vi "Do_ADAM_channel.vi"(4 "Scan Period":dbl format="%.2f", 5 "Previous Scan Value":dbl format="%.2f", 6 "Present scan array":dbl[](array[numeric]) format="%.2f", 7 "Value to Output":dbl format="%.2f", 8 "Ch Description":T1 {"Duty" format="%.0b"; "D" format="%#_5g"; "C" format="%#_5g"; "B" format="%#_5g"; "A" format="%#_5g"}, 9 "Ch names":string[](array[string])) -> (0 "Scan comment":string, 1 "Output":dbl format="%.3f")   [LabVIEW 2011]
uses:
  ADAM Client/Sub VIs/ADAM Controls/Ch_description_ADAM.ctl
  ADAM Client/Sub VIs/ADAM Controls/Module_type_ADAM.ctl
  ADAM Client/Sub VIs/ADAM Controls/Function_ADAM.ctl
  ADAM Client/Sub VIs/ADAM Controls/Channel_State.ctl
  ADAM Client/Sub VIs/ADAM Controls/Calib_type_ADAM.ctl
  ADAM Client/Sub VIs/ADAM Controls/Address.ctl
  ADAM Client/Sub VIs/ADAM Controls/Remember_value_mode.ctl
  ADAM Client/Sub VIs/ADAM Controls/Search_mode.ctl
  Anemometry/Anemometry Sub Vis/Controls/In_Range.ctl
  Anemometry/Anemometry Sub Vis/Globals/Gas_management_global.vi
  ADAM_Global.vi
  Anemometry/Anemometry Sub Vis/Globals/Constants_global.vi
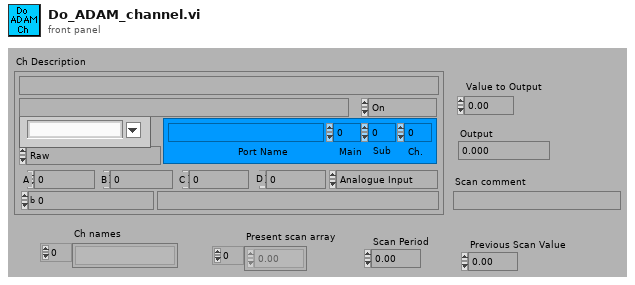
[diagram p1: front panel]
types:
  T1 = typedef "Ch_description_ADAM.ctl" = cluster{"Ch Name":string, "Type":T2, "Function":T3, "Ch State":T4, "Calibration type":T5, "A":dbl, "B":dbl, "C":dbl, "D":dbl, "Comments":string, "Address":T6, "String":string, "Duty":u16}
  T2 = typedef "Module_type_ADAM.ctl" = string
  T3 = typedef "Function_ADAM.ctl" = enum16{"Analogue Input", "Digital Input", "Event counter", "Event rate", "Analogue Output", "Digital Output", "Relay Output"}
  T4 = typedef "Channel_State.ctl" = enum16{"On", "Off", "Always On", "Always Off"}
  T5 = typedef "Calib_type_ADAM.ctl" = enum16{"Raw", "Bx + A", "Cx^2 + Bx + A", "Dx^3 + Cx^2 + Bx + A", "In Band", "Hi-Tec Q", "Hi-Tec M_dot", "Text"}
  T6 = typedef "Address.ctl" = cluster{"Main":i32, "Ch.":i32, "Sub":i32, "Port Name":string}
  T7 = typedef "Remember_value_mode.ctl" = enum16{"Read only", "Read and Write"}
  T8 = typedef "Search_mode.ctl" = enum16{"Between times", "All Times"}
  T9 = typedef "In_Range.ctl" = enum16{"%", "±", "% & ±"}
  T10 = typedef "Valco_valve_ph.ctl" = u16
  T11 = cluster{"Centre Times":dbl[], "Output array":dbl[]}
  T12 = cluster{"Centre Times":dbl[], "Output array":dbl[]}[]
  T13 = typedef "LVDateTimeRec.ctl" = cluster{"fractional second":dbl, "second":i32, "minute":i32, "hour":i32, "day of month":i32, "month":i32, "year":i32, "day of week":i32, "day of year":i32, "DST":i32}
  T14 = typedef "Client_State_Cluster.ctl" = cluster{"Client Name":string, "Traverse level State":T15, "People to Email":string[], "Next Contact Time":dbl}
  T15 = typedef "Traverse_Level_State.ctl" = enum16{"Running", "Complete"}
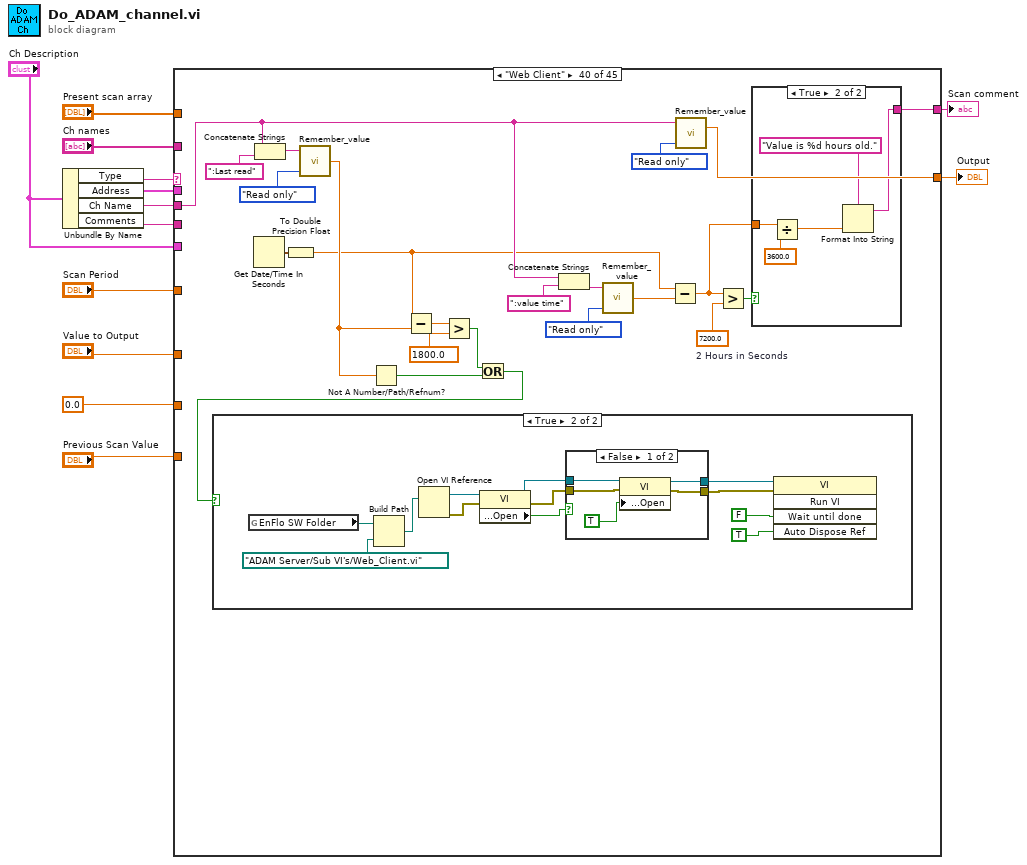
[diagram p0: block diagram]
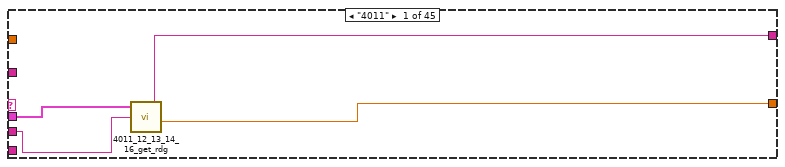
[diagram p2: hidden frame]
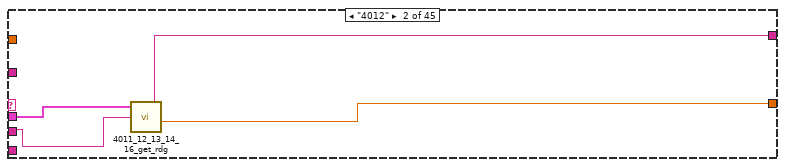
[diagram p3: hidden frame]
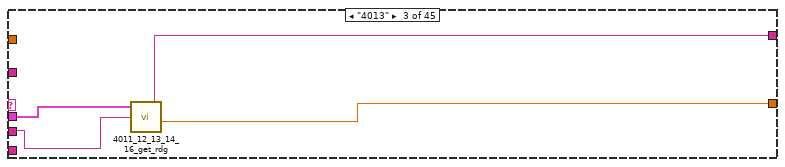
[diagram p4: hidden frame]
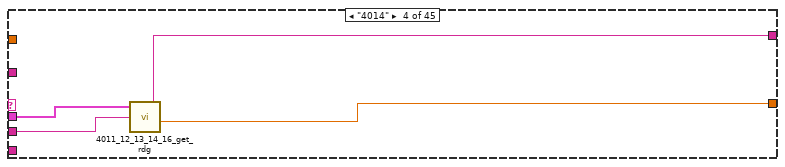
[diagram p5: hidden frame]
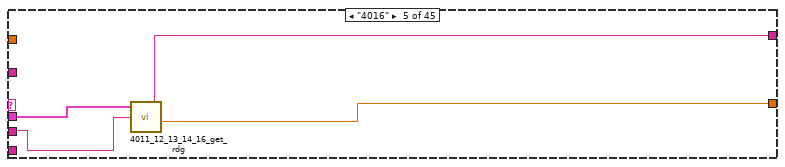
[diagram p6: hidden frame]
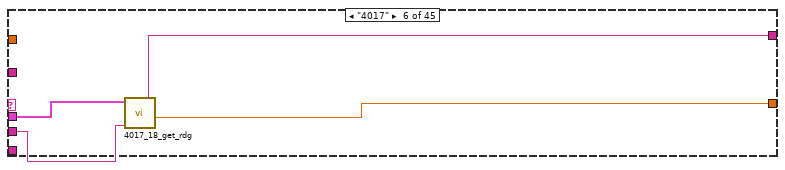
[diagram p7: hidden frame]
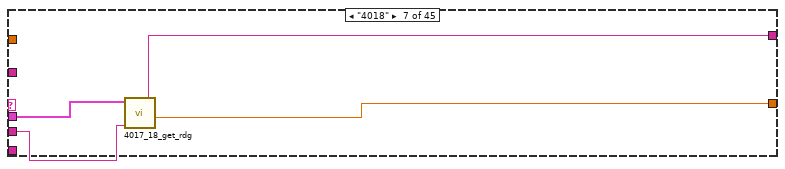
[diagram p8: hidden frame]
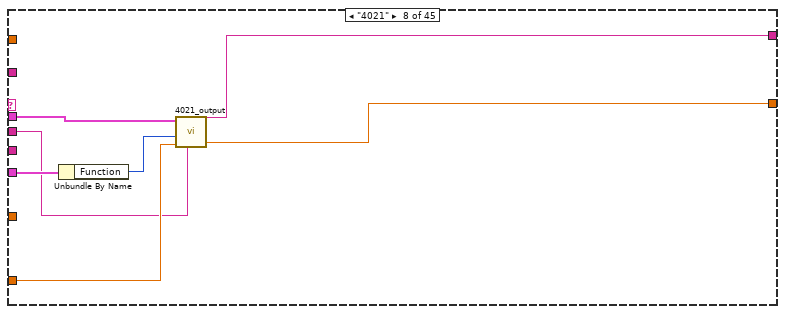
[diagram p9: hidden frame]
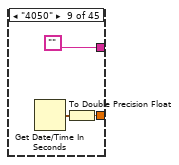
[diagram p10: hidden frame]
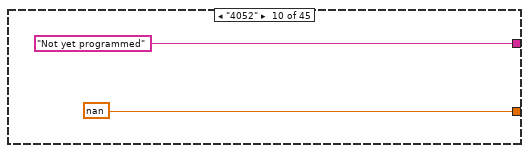
[diagram p11: hidden frame]
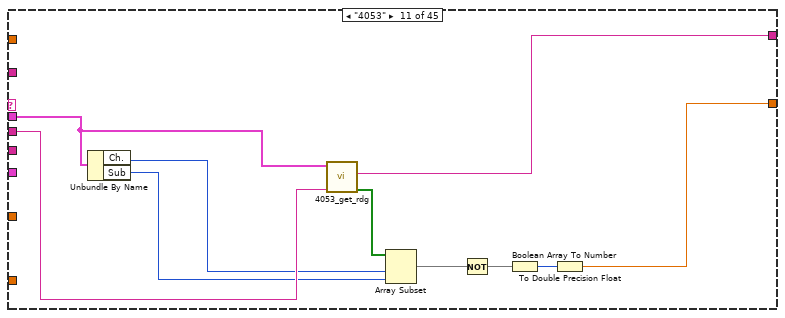
[diagram p12: hidden frame]
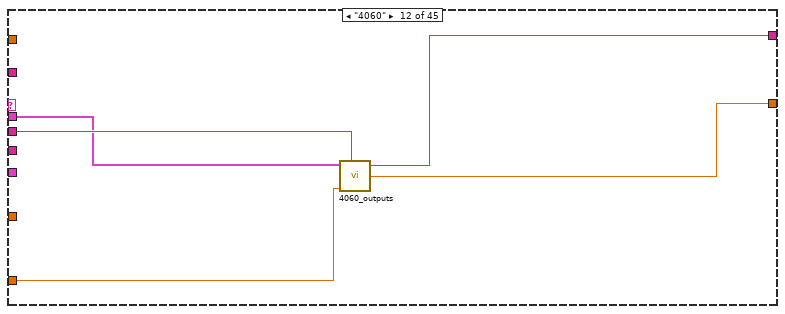
[diagram p13: hidden frame]
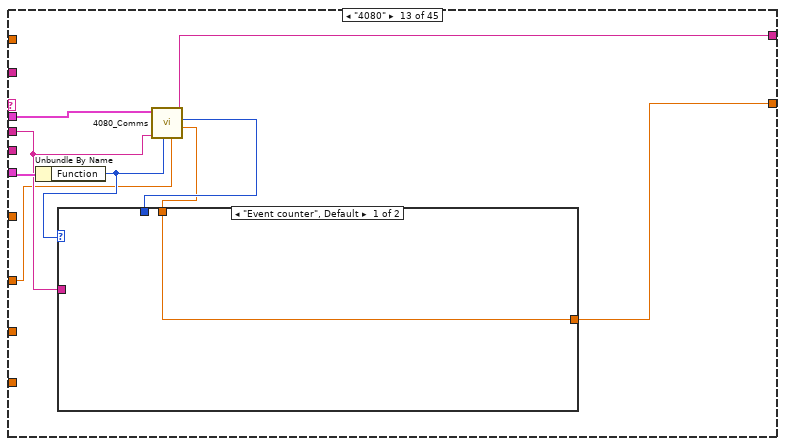
[diagram p14: hidden frame]
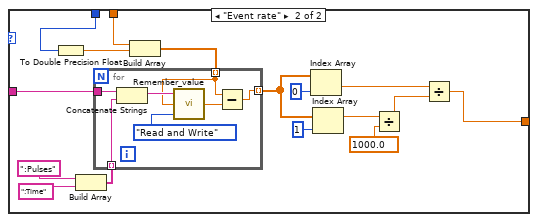
[diagram p15: hidden frame]
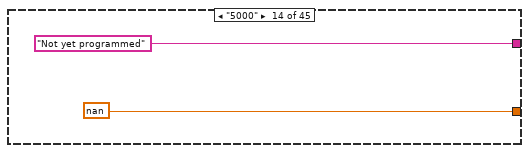
[diagram p16: hidden frame]
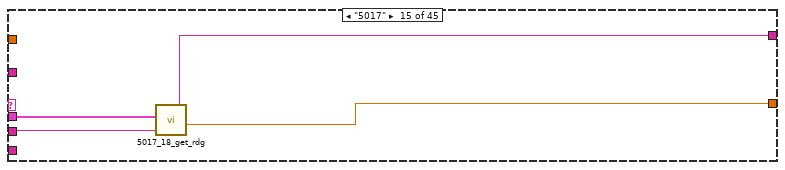
[diagram p17: hidden frame]
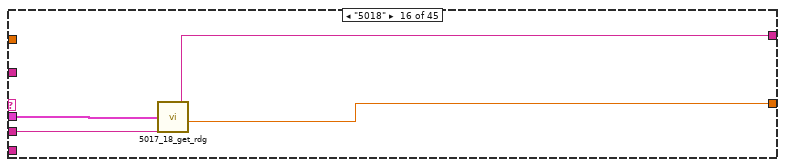
[diagram p18: hidden frame]
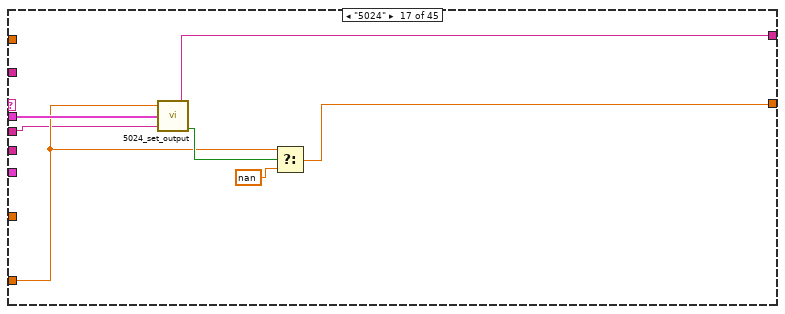
[diagram p19: hidden frame]
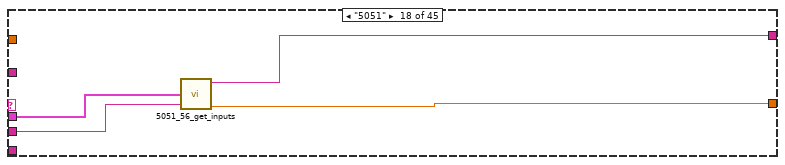
[diagram p20: hidden frame]
diagram:
  n1 = Unbundle By Name("Ch Description") -> ("Type"=w11:T2, "Address"=w10:T6, "Ch Name"=w2:string, "Comments"=w7:string)
  n2 = case shown="\"Web Client\"" w11 {
    tunnel: [w16 w20 w24 w28 w32 w36 w40 w47 w50 nan w57 w66 w75 nan w105 w109 w114 w120 w128 w149 w171 w190 nan w258 w260 w274 w299 w338 w348 w379 w384 w385 w497 w921 w923 w927 w932 nan ("Output") w946 w979 w1005 w1015 w1020 w1030 0.0 ("Output")] -> w8
    tunnel: [w17 w21 w25 w29 w33 w37 w41 w48 "" "Not yet programmed" w62 w67 w77 "Not yet programmed" w106 w110 w117 w121 w127 w150 w172 w192 "Not yet programmed" w257 w261 w273 w291 w339 w347 w380 w383 w406 w496 "" "" w928 "" "Not Yet Implemented" ("Status note") "" w968 "" w1016 w1019 "Crazy time based random number!" "Warning; unmatched case in Do_ADAM_channel" ("Status note")] -> w5
    tunnel: w10 -> [w14 w18 w22 w26 w30 w34 w38 w42 _ _ w54 w65 w69 _ w107 w111 w118 w122 w126 w151 w173 w194 _ w255 w259 w278 w296 w344 _ w378 w381 _ w488 _ _ _ _ _ _ _ w1014 w1018 _ _ _]
    tunnel: "Ch Description" -> [_ _ _ _ _ _ _ w46 _ _ _ _ w76 _ _ _ _ _ w125 w148 w170 w193 _ _ _ _ _ _ w353 _ _ w411 w490 _ w924 w929 _ _ _ _ _ _ w1021 _ _]
    tunnel: w2 -> [w15 w19 w23 w27 w31 w35 w39 w43 _ _ w63 w68 w72 _ w104 w108 w112 w119 w123 w145 w167 w191 _ w256 _ w276 w292 w343 _ _ w382 _ w493 _ _ _ _ _ w942 w975 _ w1017 _ _ _]
    tunnel: "Ch names" -> [_ _ _ _ _ _ _ _ _ _ _ _ _ _ _ _ _ _ _ _ _ _ _ _ _ _ _ _ w354 _ _ w410 w495 _ _ w930 _ _ _ _ _ _ _ _ _]
    tunnel: "Present scan array" -> [_ _ _ _ _ _ _ _ _ _ _ _ _ _ _ _ _ _ _ _ _ _ _ _ _ _ _ _ w351 _ _ w408 w494 _ _ w931 _ _ _ _ _ _ _ _ _]
    tunnel: w7 -> [_ _ _ _ _ _ _ _ _ _ _ _ _ _ _ _ _ _ _ _ _ _ _ _ _ _ _ _ w346 _ _ w412 _ _ _ _ _ _ _ _ _ _ _ _ _]
    tunnel: "Value to Output" -> [_ _ _ _ _ _ _ w44 _ _ _ w64 w70 _ _ _ w113 _ w124 w146 w168 w189 _ _ _ w262 w300 _ w352 _ _ _ _ _ _ _ _ _ _ _ w1009 _ _ _ _]
    tunnel: "Scan Period" -> [_ _ _ _ _ _ _ _ _ _ _ _ _ _ _ _ _ _ _ _ _ _ _ _ _ _ _ _ w349 _ _ _ w492 _ _ _ _ _ _ _ _ _ _ _ _]
    tunnel: "Previous Scan Value" -> [_ _ _ _ _ _ _ _ _ _ _ _ _ _ _ _ _ _ _ _ _ _ _ _ _ _ _ _ w350 _ _ w386 w491 w921 _ _ w932 _ _ _ _ _ _ _ _]
    tunnel: 0.0 -> [_ _ _ _ _ _ _ _ _ _ _ _ _ _ _ _ _ _ _ _ _ _ _ _ _ _ _ _ _ _ _ _ w489 _ _ _ _ _ _ _ _ _ _ _ _]
    frame "4011" {
      n3 = call "4011_12_13_14_16_get_rdg.vi"("Address"=w14, "Channel Name"=w15) -> ("Comment"=w17:string, "Reading"=w16:dbl)  [unwired: 1 in, 2 out]
    }
    frame "4012" {
      n4 = call "4011_12_13_14_16_get_rdg.vi"("Address"=w18, "Channel Name"=w19) -> ("Comment"=w21:string, "Reading"=w20:dbl)  [unwired: 1 in, 2 out]
    }
    frame "4013" {
      n5 = call "4011_12_13_14_16_get_rdg.vi"("Address"=w22, "Channel Name"=w23) -> ("Comment"=w25:string, "Reading"=w24:dbl)  [unwired: 1 in, 2 out]
    }
    frame "4014" {
      n6 = call "4011_12_13_14_16_get_rdg.vi"("Address"=w26, "Channel Name"=w27) -> ("Comment"=w29:string, "Reading"=w28:dbl)  [unwired: 1 in, 2 out]
    }
    frame "4016" {
      n7 = call "4011_12_13_14_16_get_rdg.vi"("Address"=w30, "Channel Name"=w31) -> ("Comment"=w33:string, "Reading"=w32:dbl)  [unwired: 1 in, 2 out]
    }
    frame "4017" {
      n8 = call "4017_18_get_rdg.vi"("Channel Name"=w35, "Address"=w34) -> ("Reading"=w36:dbl, "Comment"=w37:string)  [unwired: 2 in, 2 out]
    }
    frame "4018" {
      n9 = call "4017_18_get_rdg.vi"("Channel Name"=w39, "Address"=w38) -> ("Reading"=w40:dbl, "Comment"=w41:string)  [unwired: 2 in, 2 out]
    }
    frame "4021" {
      n10 = Unbundle By Name(w46) -> ("Function"=w45:T3)
      n11 = call "4021_output.vi"("Address"=w42, "Function"=w45, "Set to:"=w44, "Channel Name"=w43) -> ("Comment"=w48:string, "Reading"=w47:dbl)  [unwired: 1 in, 1 out]
    }
    frame "4050" {
      n12 = Get Date/Time In Seconds() -> (seconds since 1Jan1904=w49:timestamp)
      n13 = To Double Precision Float(number=w49) -> (double precision float=w50:dbl)
    }
    frame "4052" {
    }
    frame "4053" {
      n14 = Unbundle By Name(w54) -> ("Ch."=w55:i32, "Sub"=w61:i32)
      n15 = call "4053_get_rdg.vi"("Channel Name"=w63, "Address"=w54) -> ("Boolean array"=w60:bool[], "Comment"=w62:string)  [unwired: 2 in, 2 out]
      n16 = Array Subset(array=w60, index=w55, length=w61) -> (w59:bool[])
      n17 = Not(x=w59) -> (.not. x?=w56:bool[])
      n18 = Boolean Array To Number(Boolean array=w56) -> (number=w58:u32)
      n19 = To Double Precision Float(number=w58) -> (double precision float=w57:dbl)
    }
    frame "4060" {
      n20 = call "4060_outputs.vi"("Address"=w65, "Value to Output"=w64, "Channel Name"=w68) -> ("Comment"=w67:string, "Reading"=w66:dbl)  [unwired: 2 in, 1 out]
    }
    frame "4080" {
      n21 = Unbundle By Name(w76) -> ("Function"=w71:T3)
      n22 = call "4080_Comms.vi"("Value to display"=w70, "Function"=w71, "Channel Name"=w72, "Address"=w69) -> ("Reading"=w73:dbl, "millisecond timer value"=w74:u32, "Comment"=w77:string)  [unwired: 2 in, 1 out]
      n23 = case shown="\"Event counter\", Default" w71 {
        tunnel: w72 -> [_ w94]
        tunnel: w74 -> [_ w87]
        tunnel: [w78 w79] -> w75
        tunnel: w73 -> [w78 w88]
        frame "Event counter", Default {
        }
        frame "Event rate" {
          n24 = To Double Precision Float(number=w87) -> (double precision float=w86:dbl)
          n25 = Build Array(":Pulses", ":Time") -> (w89:string[])
          n26 = Build Array(w88, w86) -> (w85:dbl[])
          n27 = for {
            tunnel: w94 -> [w98]
            tunnel: [w99] -> w82 mode=indexing
            tunnel: w89 -> [w96] mode=indexing
            tunnel: w85 -> [w95] mode=indexing
            n28 = Concatenate Strings(w98, w96) -> (w97:string)
            n29 = call "Remember_value.vi"("Mode"=Remember_value_mode."Read and Write", "Input Value"=w95, "Ch name"=w97) -> ("Output Value"=w100:dbl)
            n30 = Subtract(x=w95, y=w100) -> (x-y=w99:dbl)
          }
          n31 = Index Array(array=w82, index=0) -> (element=w80:dbl)
          n32 = Index Array(array=w82, index=1) -> (element=w81:dbl)
          n33 = Divide(x=w81, y=1000.0) -> (x/y=w92:dbl)
          n34 = Divide(x=w80, y=w92) -> (x/y=w79:dbl)
        }
      }
    }
    frame "5000" {
    }
    frame "5017" {
      n35 = call "5017_18_get_rdg.vi"("Address (all reqd.)"=w107, "Channel Name"=w104) -> ("Comment"=w106:string, "Reading"=w105:dbl)  [unwired: 3 out]
    }
    frame "5018" {
      n36 = call "5017_18_get_rdg.vi"("Address (all reqd.)"=w111, "Channel Name"=w108) -> ("Comment"=w110:string, "Reading"=w109:dbl)  [unwired: 3 out]
    }
    frame "5024" {
      n37 = call "5024_set_output.vi"("Set to:"=w113, "Address (all reqd.)"=w118, "Channel Name"=w112) -> ("Comment"=w117:string, "Good Reply"=w115:bool)  [unwired: 2 out]
      n38 = Select(t=w113, s=w115, f=nan) -> (s? t:f=w114:dbl)
    }
    frame "5051" {
      n39 = call "5051_56_get_inputs.vi"("Address (Main, Sub reqd.)"=w122, "Channel Name"=w119) -> ("Comment"=w121:string, "Single output"=w120:dbl)  [unwired: 3 out]
    }
    frame "5056" {
      n40 = Unbundle By Name(w125) -> ("Function"=w129:T3)
      n41 = case shown="\"Digital Input\"" w129 {
        tunnel: w126 -> [_ w135 w144]
        tunnel: ["This function is not available" w136 w142] -> w127
        tunnel: [nan ("A") w133 w139] -> w128
        tunnel: w124 -> [_ _ w138]
        tunnel: w123 -> [_ w132 w137]
        frame "Analogue Input", Default {
        }
        frame "Digital Input" {
          # "Readback value"
          n42 = call "5060_check_outputs.vi"("Address (Main, Sub reqd.)"=w135, "Channel Name"=w132) -> ("Comment"=w136:string, "Single Channel"=w134:i16)  [unwired: 3 out]
          n43 = To Double Precision Float(number=w134) -> (double precision float=w133:dbl)
        }
        frame "Relay Output" {
          # "Sets single o/p channel"
          n44 = Greater Than 0?(x=w138) -> (x > 0?=w143:bool)
          n45 = call "5056_60_set_single_output.vi"("Channel Name"=w137, "Address (all reqd.)"=w144, "Set state:"=w143) -> ("Comment"=w142:string, "Good Reply"=w141:bool)  [unwired: 2 out]
          n46 = Select(t=w138, s=w141, f=nan) -> (s? t:f=w139:dbl)
        }
      }
    }
    frame "5060" {
      n47 = Unbundle By Name(w148) -> ("Function"=w147:T3)
      n48 = case shown="\"Relay Output\"" w147 {
        tunnel: w151 -> [_ w157 w166]
        tunnel: ["This function is not available" w158 w164] -> w150
        tunnel: [nan ("A") w155 w161] -> w149
        tunnel: w146 -> [_ _ w160]
        tunnel: w145 -> [_ w154 w159]
        frame "Analogue Input", Default {
        }
        frame "Digital Input" {
          # "Readback value"
          n49 = call "5060_check_outputs.vi"("Address (Main, Sub reqd.)"=w157, "Channel Name"=w154) -> ("Comment"=w158:string, "Single Channel"=w156:i16)  [unwired: 3 out]
          n50 = To Double Precision Float(number=w156) -> (double precision float=w155:dbl)
        }
        frame "Relay Output" {
          # "Sets single o/p channel"
          n51 = Greater Than 0?(x=w160) -> (x > 0?=w165:bool)
          n52 = call "5056_60_set_single_output.vi"("Channel Name"=w159, "Address (all reqd.)"=w166, "Set state:"=w165) -> ("Comment"=w164:string, "Good Reply"=w163:bool)  [unwired: 2 out]
          n53 = Select(t=w160, s=w163, f=nan) -> (s? t:f=w161:dbl)
        }
      }
    }
    frame "6060" {
      n54 = Unbundle By Name(w170) -> ("Function"=w169:T3)
      n55 = case shown="\"Digital Input\"" w169 {
        tunnel: w173 -> [_ w179 w188]
        tunnel: ["This function is not available" w180 w186] -> w172
        tunnel: [nan ("A") w177 w183] -> w171
        tunnel: w168 -> [_ _ w182]
        tunnel: w167 -> [_ w176 w181]
        frame "Analogue Input", Default {
        }
        frame "Digital Input" {
          n56 = call "6060_read_all_I-O.vi"("Address (Main, Sub reqd.)"=w179, "Channel Name"=w176) -> ("Comment"=w180:string, "Single Input Channel"=w178:i16)  [unwired: 3 out]
          n57 = To Double Precision Float(number=w178) -> (double precision float=w177:dbl)
        }
        frame "Relay Output" {
          # "Sets single o/p channel"
          n58 = Greater Than 0?(x=w182) -> (x > 0?=w187:bool)
          n59 = call "6060_set_single_output.vi"("Channel Name"=w181, "Address (Main, Ch requd.)"=w188, "Set state:"=w187) -> ("Comment"=w186:string, "Good Reply"=w185:bool)  [unwired: 2 out]
          n60 = Select(t=w182, s=w185, f=nan) -> (s? t:f=w183:dbl)
        }
      }
    }
    frame "Tracker" {
      n61 = while {
        tunnel: w194 -> [w218]
        tunnel: w193 -> [w217]
        tunnel: [w211] -> w192
        tunnel: w191 -> [w210]
        tunnel: [w204] -> w190
        tunnel: w189 -> [w203]
        i -> [w200]
        stop <- w197 continue-if-true
        n62 = Unbundle By Name(w217) -> ("Function"=w216:T3)
        n63 = Unbundle By Name(w218) -> ("Port Name"=w215:string, "Ch."=w206:i32, "Main"=w214:i32, "Sub"=w213:i32)
        n64 = case shown="\"Analogue Output\"" w216 {
          tunnel: [enum16{"Set", "Read"}."Set" ("Set") enum16{"Set", "Read"}."Set" ("Set") enum16{"Set", "Read"}."Set" ("Set") enum16{"Set", "Read"}."Set" ("Set") enum16{"Set", "Read"}."Set" ("Set") enum16{"Set", "Read"}."Read" ("Set") enum16{"Set", "Read"}."Read" ("Set")] -> w201
          tunnel: [enum16{"Logic", "Analogue"}."Analogue" ("Analogue") enum16{"Logic", "Analogue"}."Logic" ("Analogue") enum16{"Logic", "Analogue"}."Logic" ("Analogue") enum16{"Logic", "Analogue"}."Logic" ("Analogue") enum16{"Logic", "Analogue"}."Logic" ("Analogue") enum16{"Logic", "Analogue"}."Logic" ("Analogue") enum16{"Logic", "Analogue"}."Analogue" ("Analogue")] -> w212
          frame "Analogue Output" {
          }
          frame "Digital Output" {
          }
          frame "Relay Output" {
          }
          frame "Event rate" {
          }
          frame "Event counter" {
          }
          frame "Digital Input" {
          }
          frame "Analogue Input" {
          }
        }
        n65 = call "TalkTracker.vi"("PORT NAME"=w215, "Set"=w201, "Channel Name"=w210, "Value to set"=w203, "MODULE ADDRESS"=w214, "LOCATION"=w206, "NO. LOCATIONS"=w213, "Analogue"=w212) -> ("Response"=w208:string, "Good Set?"=w195:bool, "Comment out"=w211:string)  [unwired: 1 in, 4 out]
        n66 = Match Pattern(string=w208, regular expression="\r\n") -> (before substring=w207:string)  [unwired: 4 out]
        n67 = case shown="\"Set\"" w201 {
          tunnel: w207 -> [_ w230]
          tunnel: [w222 w229] -> w205
          tunnel: w203 -> [w224 _]
          tunnel: nan ("Reading") -> [w223 w228]
          tunnel: [w221 w226] -> w198
          tunnel: [0 ("y") 1 ("y")] -> w196
          tunnel: w195 -> [w219 _]
          frame "Set" {
            n68 = Not(x=w219) -> (.not. x?=w221:bool)
            n69 = Select(t=w224, s=w219, f=w223) -> (s? t:f=w222:dbl)
          }
          frame "Read" {
            n70 = String Length(string=w230) -> (length=w232:i32)
            n71 = Fract/Exp String To Number(string=w230, default (0 dbl)=w228) -> (offset past number=w233:i32, number=w231:dbl)  [unwired: 2 out]
            n72 = Equal?(x=w232, y=w233) -> (x = y?=w227:bool)
            n73 = Not(x=w227) -> (.not. x?=w226:bool)
            n74 = Select(t=w231, s=w227, f=w228) -> (s? t:f=w229:dbl)
          }
        }
        n75 = case shown="0, Default" w206 {
          tunnel: w205 -> [w234 w237]
          tunnel: [w234 w235] -> w204
          frame 0, Default {
          }
          frame 283 {
            n76 = Equal To 0?(x=w237) -> (x = 0?=w238:bool)
            n77 = Select(t=nan ("Reading"), s=w238, f=w237) -> (s? t:f=w235:dbl)
          }
        }
        n78 = Less?(x=w200, y=w196) -> (x < y?=w199:bool)
        n79 = And(x=w198, y=w199) -> (x .and. y?=w197:bool)
      }
    }
    frame "WEST" {
    }
    frame "GILL" {
      n80 = call "Gill_get_rdg.vi"("Channel Name"=w256, "Address"=w255) -> ("Output"=w258:dbl, "Status note"=w257:string)  [unwired: 2 in, 2 out]
    }
    frame "ClimatronicsUDP" {
      n81 = call "ClimatronicsUDP_get_rdg.vi"("Address"=w259) -> ("Output"=w260:dbl, "Status note"=w261:string)  [unwired: 5 in]
    }
    frame "JEM" {
      n82 = Unbundle By Name(w278) -> ("Main"=w265:i32, "Ch."=w264:i32, "Port Name"=w277:string)
      n83 = case shown="0, Default" w264 {
        tunnel: [i16[] [-3, -2, -1, 0, 14, 29, 43, 57, 71, 86, 100] i16[] [0, 20, 40, 60, 80, 100, 120]] -> w268
        tunnel: [u8[] [10, 50, 80, 100, 120, 140, 160, 180, 200, 220, 240] u8[] [20, 50, 90, 130, 160, 200, 230]] -> w269
        frame 0, Default {
        }
        frame 1 {
        }
      }
      n84 = Add(x=w265, y=w264) -> (x+y=w263:i32)
      n85 = Threshold 1D Array(2:w262, 3:w268) -> (0:w271:dbl)  [unwired: 1 out]
      n86 = Round To Nearest(number=w271) -> (nearest integer value=w272:dbl)
      n87 = To Long Integer(number=w272) -> (32bit integer=w270:i32)
      n88 = Index Array(array=w269, index=w270) -> (element=w267:u8)
      n89 = call "DMX.vi"("Port Name"=w277, "DMX channel no."=w263, "Set value:"=w267, "Channel Name"=w276) -> ("error"=w275:bool)  [unwired: 2 out]
      n90 = Index Array(array=w268, index=w270) -> (element=w266:i16)
      n91 = case shown="False" w275 {
        tunnel: [w279 nan] -> w274
        tunnel: ["" "Comms Error"] -> w273
        tunnel: w266 -> [w281 _]
        frame False {
          n92 = To Double Precision Float(number=w281) -> (double precision float=w279:dbl)
        }
        frame True {
        }
      }
    }
    frame "VICI" {
      n93 = To Long Integer(number=w300) -> (32bit integer=w295:i32)
      n94 = Unbundle By Name(w296) -> ("Port Name"=w298:string, "Ch."=w297:i32)
      n95 = call "Valco_Valve_Position.vi"("Channel Name"=w292, "Valve Number"=w297, "Port Name"=w298, "Requested Posn."=w295) -> ("Error Message"=w290:string, "Achieved Posn."=w293:T10)  [unwired: 2 out]
      n96 = Empty String/Path?(string/path=w290) -> ()  [unwired: 1 out]
      n97 = case shown="True" TRUE {
        tunnel: w296 -> [w307 _]
        tunnel: w295 -> [w306 _]
        tunnel: [w305 w337] -> w294
        tunnel: w293 -> [_ w337]
        tunnel: w292 -> [w304 _]
        tunnel: [w303 w336] -> w291
        tunnel: w290 -> [_ w336]
        tunnel: w290 -> [w302 _]
        tunnel: "X10" ("Port Name") -> [w301 _]
        frame False {
          n98 = stacked-sequence {
            tunnel: w307 -> [_ _ _ _ _ w328]
            tunnel: w306 -> [_ _ _ _ _ w324]
            tunnel: [_ _ _ _ _ w327] -> w305
            tunnel: w304 -> [_ _ _ _ _ w326]
            tunnel: [_ _ _ _ _ w325] -> w303
            tunnel: w302 -> [_ w313 _ _ _ _]
            tunnel: w301 -> [w308 _ _ w316 _ _]
            frame #0 {
              w310 = 3 items=["-----", "A", "B", "C", "D", "E", "F", "G", "H", "I", "J", "K", "L", "M", "N", "O", "P"] ("House Code")
              n99 = call "X10control.vi"("Port Name"=w308, "Power Request (ON)"=FALSE, "House Code"=w310, "Unit No."=5) -> ()  [unwired: 6 out]
            }
            frame #1 {
              n100 = call "Server_Emails.vi"("Message"=w313, "Contact All clients?"=TRUE, "Subject"="Powering Down FID Valve" ("Error Type")) -> ()  [unwired: 2 in, 3 out]
            }
            frame #2 {
              n101 = Wait (ms)(milliseconds to wait=u32 20000) -> ()  [unwired: 1 out]
            }
            frame #3 {
              w318 = 3 items=["-----", "A", "B", "C", "D", "E", "F", "G", "H", "I", "J", "K", "L", "M", "N", "O", "P"] ("House Code")
              n102 = call "X10control.vi"("Port Name"=w316, "Power Request (ON)"=TRUE, "House Code"=w318, "Unit No."=5) -> ()  [unwired: 6 out]
            }
            frame #4 {
              n103 = Wait (ms)(milliseconds to wait=u32 5000) -> ()  [unwired: 1 out]
            }
            frame #5 {
              n104 = Build Array(1 ("element"), 2 ("element"), w324) -> (w321:i32[])
              n105 = for {
                tunnel: w328 -> [w333]
                tunnel: [w332] -> w327
                tunnel: w326 -> [w331]
                tunnel: [w330] -> w325
                tunnel: w321 -> [w329] mode=indexing
                n106 = Unbundle By Name(w333) -> ("Port Name"=w334:string, "Ch."=w335:i32)
                n107 = call "Valco_Valve_Position.vi"("Channel Name"=w331, "Valve Number"=w335, "Port Name"=w334, "Requested Posn."=w329) -> ("Error Message"=w330:string, "Achieved Posn."=w332:T10)  [unwired: 2 out]
              }
            }
          }
        }
        frame True {
        }
      }
      n108 = To Double Precision Float(number=w294) -> (double precision float=w299:dbl)
    }
    frame "Vaisala" {
      n109 = Unbundle By Name(w344) -> ("Main"=w340:i32, "Ch."=w341:i32, "Port Name"=w342:string)
      n110 = call "HMP231.vi"("Channel Name"=w343, "Port Name"=w342, "Channel"=w341, "Address"=w340) -> ("Output"=w338:dbl, "Status note"=w339:string)  [unwired: 2 out]
    }
    frame "Run VI Named:" {
      n111 = Current VI's Path() -> (path=w363:path)
      n112 = Strip Path(path=w363) -> (stripped path=w364:path)  [unwired: 1 out]
      n113 = call <vilib>:"Trim Whitespace.vi"("string"=w346) -> ("trimmed string"=w345:string)  [unwired: 1 in]
      n114 = Strip Path(path=w364) -> (stripped path=w365:path)  [unwired: 1 out]
      n115 = Build Path(base path=w365, name or relative path="Run_vi_named") -> (appended path=w367:path)
      n116 = Build Path(base path=w367, name or relative path=w345) -> (appended path=w362:path)
      n117 = Open VI Reference(type specifier VI Refnum (for type only)=refnum<vi> refnum, vi path=w362) -> (vi reference=w358:refnum<vi>, error out=w357:errorcluster)  [unwired: 1 in, 3 out]
      n118 = property class="VI Interface Type 7"(reference=w358, error in=w357) -> (reference out=w360:refnum<vi>, error out=w359:errorcluster, "Front Panel Window:Open"=w361:bool)
      n119 = case shown="False" w361 {
        tunnel: w360 -> [w375 w377]
        tunnel: w359 -> [w374 w376]
        tunnel: [w373 w377] -> w356
        tunnel: [w371 w376] -> w355
        frame False {
          n120 = property class="VI Interface Type 7"(reference=w375, error in=w374, "Front Panel Window:Open"=TRUE) -> (reference out=w373:refnum<vi>, error out=w371:errorcluster)
        }
        frame True {
        }
      }
      n121 = call-by-ref "?"(reference=w356, error in=w355, "Scan Period"=w349, "Previous Scan Value"=w350, "Present scan array"=w351, "Value to Output"=w352, "Ch Description"=w353, "Ch names"=w354) -> (reference out=w369:refnum<vi>, error out=w370:errorcluster, "Scan comment"=w347:string, "Output"=w348:dbl)  [unwired: 2 in]
      n122 = Close Reference(reference=w369, error in (no error)=w370) -> ()  [unwired: 1 out]
    }
    frame "IR2100" {
      n123 = call "IR2100_get_rdg.vi"("Address"=w378) -> ("Comment"=w380:string, "Reading"=w379:dbl)  [unwired: 2 in, 2 out]
    }
    frame "PPT" {
      n124 = call "PPT_get_rdg.vi"("Channel Name"=w382, "Address"=w381) -> ("Reading"=w384:dbl, "Comment"=w383:string)  [unwired: 2 in, 2 out]
    }
    frame "Comparator" {
      # "A Warn if above this value\nB Warn if below this value\nC  Hysteresis margin\nD is the averaging time in minutes\nComments   is Channel name to check"
      n125 = Unbundle By Name(w411) -> ("D"=w394:dbl)
      n126 = Match Pattern(string=w412, regular expression=":::" ("String to match")) -> (before substring=w409:string)  [unwired: 4 out]
      n127 = call "Read_value_of_earlier_Ch.vi"("Desired Ch to Read"=w409, "Ch names"=w410, "Present scan array"=w408) -> ("Value"=w393:dbl, "Scan comment"=w407:string)  [unwired: 1 in]
      n128 = Equal?(x=w386, y=1.0) -> (x = y?=w402:bool)
      n129 = Unbundle By Name(w411) -> ("A"=w405:dbl, "B"=w404:dbl, "C"=w403:dbl)
      n130 = Equal To 0?(x=w394) -> (x = 0?=w392:bool)
      n131 = case shown="True" w402 {
        tunnel: [w418 w423] -> w400
        tunnel: w405 -> [w418 w422]
        tunnel: w404 -> [w417 w421]
        tunnel: [w417 w419] -> w401
        tunnel: w403 -> [_ w420]
        frame False {
        }
        frame True {
          n132 = Subtract(x=w422, y=w420) -> (x-y=w423:dbl)
          n133 = Add(x=w421, y=w420) -> (x+y=w419:dbl)
        }
      }
      n134 = case shown="False" w392 {
        tunnel: [w428 w431] -> w415
        tunnel: w409 -> [w430 _]
        tunnel: [w426 w432] -> w391
        tunnel: w394 -> [w424 _]
        tunnel: w393 -> [_ w432]
        tunnel: w407 -> [w428 w431]
        frame False {
          n135 = Build Array(w430) -> (w425:string[])
          n136 = call "Get_Channel_averages.vi"("Desired Ch Names"=w425, "Averaging time (mins)"=w424) -> ("number"=w427:dbl[])  [unwired: 1 in, 2 out]
          n137 = Index Array(array=w427, index=0) -> (element=w426:dbl)
        }
        frame True {
        }
      }
      n138 = Not(x=w402) -> (.not. x?=w395:bool)
      n139 = In Range and Coerce(upper limit=w400, x=w391, lower limit=w401) -> (In Range?=w396:bool)  [unwired: 1 out]
      n140 = Greater?(x=w391, y=w400) -> (0:w399:bool)
      n141 = Not A Number/Path/Refnum?(number/path/refnum=w391) -> (NaN/Path/Refnum?=w388:bool)
      n142 = Equal?(x=w396, y=w395) -> (x = y?=w390:bool)
      n143 = Or(x=w390, y=w388) -> (x .or. y?=w389:bool)
      n144 = case shown="False" w389 {
        tunnel: w409 -> [w439 _]
        tunnel: w400 -> [w438 _]
        tunnel: w411 -> [w437 _]
        tunnel: w401 -> [w436 _]
        tunnel: w396 -> [w435 _]
        tunnel: w391 -> [w434 _]
        tunnel: w399 -> [w433 _]
        frame False {
          n145 = stacked-sequence {
            seq-local: [w445 _ _ _ _] -> [_ _ _ w486 _]
            seq-local: [_ w465 _ _ _] -> [_ _ _ w483 _]
            seq-local: [w443 _ _ _ _] -> [_ _ _ w479 _]
            tunnel: w439 -> [w447 w473 _ w485 _]
            tunnel: w438 -> [w446 _ _ _ _]
            tunnel: w437 -> [_ _ w478 w487 _]
            tunnel: w436 -> [w444 _ _ _ _]
            tunnel: w435 -> [w442 _ _ _ _]
            tunnel: w434 -> [w441 _ _ _ _]
            tunnel: w433 -> [w440 _ _ _ _]
            frame #0 {
              n146 = case shown="True" w442 {
                tunnel: w447 -> [w452 w463]
                tunnel: w446 -> [_ w456]
                tunnel: [w450 w462] -> w445
                tunnel: w444 -> [_ w455]
                tunnel: ["OK " ""] -> w443
                tunnel: w441 -> [w448 _]
                tunnel: w440 -> [_ w453]
                frame True {
                  n147 = Format Into String(format string="The channel named %s is now  %.3f" ("Format String"), w452, w448) -> (resulting string=w450:string)  [unwired: 2 in, 1 out]
                }
                frame False {
                  n148 = Select(t=w456, s=w453, f=w455) -> (s? t:f=w454:dbl)
                  n149 = Select(t="greater", s=w453, f="less") -> (s? t:f=w458:string)
                  n150 = Format Into String(format string="%s is %s than %.3f" ("Format String"), w463, w458, w454) -> (resulting string=w462:string)  [unwired: 2 in, 1 out]
                }
              }
            }
            frame #1 {
              n151 = Build Array(w473) -> (w472:string[])
              n152 = call "Channel_Names_and_indicies.vi"("All Active Channels"=FALSE, "Desired Ch Names"=w472) -> ("Indicies"=w470:i32[])  [unwired: 1 out]
              n153 = call "Specified_Channels_server.vi"("Mode"=Search_mode."All Times", "Requested channels"=w470) -> ("Output array"=w468:dbl[][], "Centre Times"=w464:dbl[])  [unwired: 3 in, 3 out]
              n154 = Index Array(array=w468, index (row)=0) -> (element=w466:dbl[])  [unwired: 1 in]
              n155 = Bundle("Centre Times"=w464, "Output array"=w466) -> (w469:T11)  [unwired: 1 out]
              n156 = Build Array(w469) -> (w465:T12)
            }
            frame #2 {
              w476 = TRUE  # Contact All clients?
              n157 = Unbundle By Name(w478) -> ("String"=w477:string)
              n158 = call "Get_array_values_fr_String.vi"("String Value"=w477) -> ("String array"=w475:string[])  [unwired: 1 out]
              n159 = call "Client_email_addresses.vi"("Extra People to Email"=w475, "Contact All clients?"=w476) -> ()  [unwired: 1 in]
            }
            frame #3 {
              n160 = Unbundle By Name(w487) -> ("Ch Name"=w480:string)
              n161 = Build Array(w485) -> (w484:string[])
              n162 = Concatenate Strings(w479, w480) -> (w481:string)
              n163 = call "Email_Attachment_Plot.vi"("X axis name"="Time", "XY Graph"=w483, "Series Names"=w484, "message"=w486, "subject ([No Subject])"=w481) -> ()  [unwired: 1 in, 1 out]
            }
            frame #4 {
            }
          }
        }
        frame True {
        }
      }
      n164 = Concatenate Strings(w415, "") -> (w406:string)
      n165 = Select(t=0.0, s=w396, f=1.0) -> (s? t:f=w387:dbl)
      n166 = Select(t=w386, s=w388, f=w387) -> (s? t:f=w385:dbl)
    }
    frame "VIRTUAL" {
      n167 = case shown="\"Laser:Cooling_Water:Delta_T\"" w493 {
        tunnel: [w507 w521 w535 w557 w572 w583 w599 w630 w657 w692 w701 w718 w771 w797 w824 w844] -> w497
        tunnel: [w498 w527 w533 w561 w566 w581 w608 "" w661 w686 w695 w715 w770 w796 "" w845] -> w496
        tunnel: w495 -> [w504 w529 w539 w563 w568 w586 w610 w634 w663 w688 w697 w716 w776 w801 _ w847]
        tunnel: w494 -> [w505 w528 w540 w562 w567 w587 w609 w635 w664 w687 w696 w717 w778 w803 _ w846]
        tunnel: w493 -> [w502 _ _ _ _ _ _ _ _ _ _ w704 _ _ w819 _]
        tunnel: w492 -> [w503 _ _ _ _ _ _ _ _ _ _ _ w768 w795 w824 w843]
        tunnel: w491 -> [w506 _ _ _ _ _ _ _ _ _ _ w719 w772 w798 _ w842]
        tunnel: w490 -> [_ _ w531 _ _ _ _ _ _ _ _ w710 _ _ _ _]
        tunnel: w489 -> [_ w520 _ _ _ w580 _ _ _ _ _ _ _ _ _ _]
        tunnel: w488 -> [_ _ _ _ _ _ _ _ _ _ _ _ _ _ _ _]
        frame "GMU:Remaining:", Default {
          n168 = Match Pattern(string=w502, regular expression="GMU:Remaining:" ("String to match")) -> (match substring=w500:string)  [unwired: 4 out]
          n169 = Empty String/Path?(string/path=w500) -> (empty?=w499:bool)
          n170 = case shown="False" w499 {
            tunnel: [w514 nan] -> w507
            tunnel: w506 -> [w513 _]
            tunnel: w505 -> [w512 _]
            tunnel: w504 -> [w511 _]
            tunnel: w503 -> [w510 _]
            tunnel: w502 -> [w509 _]
            tunnel: [w508 w516] -> w498
            frame False {
              n171 = call "Update_Rem_gas.vi"("Scan Period (s)"=w510, "Gas Remaining in"=w513, "Ch name"=w509, "Ch names"=w511, "Present scan array"=w512) -> ("Gas Remaining out"=w514:dbl, "Comments"=w508:string)  [unwired: 1 out]
            }
            frame True {
              n172 = Current VI's Path() -> (path=w518:path)
              n173 = Path To String(path=w518) -> (string=w517:string)
              n174 = Concatenate Strings(" was not matched in ", w517) -> (w516:string)
            }
          }
        }
        frame "GMU:Source:Meas Q" {
          n175 = call "Calculate_Release_Flowrates.vi"("Ch names"=w529, "Units"=enum16{"Q l/min", "M_dot Kg/min"}."Q l/min", "Present scan array"=w528) -> ("Trace"=w525:dbl, "Carrier"=w526:dbl, "Scan comments"=w527:string)
          n176 = Add(x=w526, y=w525) -> (x+y=w522:dbl)
          n177 = Not Equal To 0?(x=w522) -> (x != 0?=w523:bool)
          n178 = Select(t=w522, s=w523, f=w520) -> (s? t:f=w521:dbl)
        }
        frame "GMU:Detector:Strength" {
          n179 = Unbundle By Name(w531) -> ("C"=w530:dbl)
          n180 = call "Read_value_of_earlier_Ch.vi"("Desired Ch to Read"="GMU:Detector:Meas Current", "Ch names"=w539, "Present scan array"=w540) -> ("Value"=w536:dbl, "Scan comment"=w534:string)  [unwired: 1 in]
          n181 = Greater?(x=w536, y=w530) -> (0:w537:bool)
          n182 = case shown="True" w537 {
            tunnel: w531 -> [_ w552]
            tunnel: w536 -> [_ w547]
            tunnel: [100.0 ("Eng Values") w545] -> w535
            tunnel: ["Fault" w548] -> w532
            frame False {
            }
            frame True {
              n183 = Unbundle By Name(w552) -> ("D"=w543:dbl, "A"=w551:dbl, "B"=w550:dbl)
              n184 = Less?(x=w547, y=w543) -> (x < y?=w546:bool)
              n185 = Build Array(w551, w550) -> (w549:dbl[])
              n186 = call "Polynomial_convert.vi"("Calib constants"=w549, "Voltage"=w547) -> ("Eng Values"=w544:dbl)  [unwired: 4 out]
              n187 = case shown="True" w546 {
                tunnel: ["Saturated" ""] -> w548
                tunnel: [100.0 ("Eng Values") w555] -> w545
                tunnel: w544 -> [_ w555]
                frame False {
                }
                frame True {
                }
              }
            }
          }
          n188 = Concatenate Strings(w534, w532) -> (w533:string)
        }
        frame "GMU:Source:Meas M_dot" {
          n189 = call "Calculate_Release_Flowrates.vi"("Ch names"=w563, "Units"=enum16{"Q l/min", "M_dot Kg/min"}."M_dot Kg/min", "Present scan array"=w562) -> ("Trace"=w559:dbl, "Carrier"=w560:dbl, "Scan comments"=w561:string)
          n190 = Add(x=w560, y=w559) -> (x+y=w557:dbl)
        }
        frame "GMU:Source:Meas Density" {
          n191 = Build Array("GMU:Source:Meas M_dot", "GMU:Source:Meas Q") -> (w569:string[])
          n192 = call "Read_Earlier_Channels.vi"("Present scan array"=w567, "Ch names"=w568, "Desired Channels"=w569) -> ("Scan comments"=w566:string, "Index 0"=w565:dbl, "Index 1"=w564:dbl)  [unwired: 3 out]
          n193 = Not Equal To 0?(x=w565) -> (x != 0?=w573:bool)
          n194 = case shown="False" w573 {
            tunnel: w565 -> [_ w577]
            tunnel: w564 -> [_ w576]
            tunnel: [0.0 w575] -> w572
            frame False {
            }
            frame True {
              n195 = Divide(x=w577, y=w576) -> (x/y=w578:dbl)
              n196 = Multiply(x=w578, y=1000.0) -> (x*y=w575:dbl)
            }
          }
        }
        frame "GMU:Source:Meas Den Ratio" {
          n197 = call "Read_value_of_earlier_Ch.vi"("Desired Ch to Read"="GMU:Source:Meas Density", "Ch names"=w586, "Present scan array"=w587) -> ("Value"=w582:dbl, "Scan comment"=w581:string)  [unwired: 1 in]
          n198 = Equal?(x=w582, y=w580) -> (x = y?=w584:bool)
          n199 = case shown="False" w584 {
            tunnel: w582 -> [w589 _]
            tunnel: [w588 w594] -> w583
            tunnel: w580 -> [_ w594]
            frame False {
              n200 = global read "Gas_management_global.vi" "Release temp (deg C)"() -> (w592:dbl)
              n201 = global read "Gas_management_global.vi" "Atmos Pres (mbars)"() -> (w591:dbl)
              n202 = call "Gas_Density.vi"("Pressure (mbars)"=w591, "Temperature (deg C)"=w592, "Gas Name"="Air") -> ("Density Kg/m3"=w590:dbl)
              n203 = Divide(x=w589, y=w590) -> (x/y=w588:dbl)
            }
            frame True {
            }
          }
        }
        frame "GMU:Source:Meas Strength" {
          n204 = call "Calculate_Release_Flowrates.vi"("Ch names"=w610, "Units"=enum16{"Q l/min", "M_dot Kg/min"}."Q l/min", "Present scan array"=w609) -> ("Trace"=w602:dbl, "Carrier"=w603:dbl, "Scan comments"=w608:string)
          n205 = Equal To 0?(x=w603) -> (x = 0?=w605:bool)
          n206 = Equal To 0?(x=w602) -> (x = 0?=w606:bool)
          n207 = And(x=w605, y=w606) -> (x .and. y?=w604:bool)
          n208 = case shown="False" w604 {
            tunnel: w603 -> [w621 _]
            tunnel: w602 -> [w620 _]
            tunnel: [w619 0.0] -> w598
            frame False {
              n209 = Add(x=w621, y=w620) -> (x+y=w624:dbl)
              n210 = Divide(x=w620, y=w624) -> (x/y=w623:dbl)
              n211 = Multiply(x=w623, y=100.0) -> (x*y=w619:dbl)
            }
            frame True {
            }
          }
          n212 = while {
            tunnel: [w612] -> w595
            tunnel: [w613] -> w597
            tunnel: w598 -> [w618]
            shift-left: _ -> [w612]
            shift-left: _ -> [w617]
            shift-right: [w618] -> _
            stop <- FALSE continue-if-true
            w616 = 6.0 ("y")
            n213 = Less?(x=w617, y=w616) -> (x < y?=w615:bool)
            n214 = Less?(x=w612, y=w616) -> (x < y?=w614:bool)
            n215 = Or(x=w615, y=w614) -> (x .or. y?=w613:bool)
          }
          n216 = Greater?(x=w598, y=7.0) -> (0:w596:bool)
          n217 = And(x=w597, y=w596) -> (x .and. y?=w600:bool)
          n218 = Select(t=w595, s=w600, f=w598) -> (s? t:f=w599:dbl)
        }
        frame "EnFlo_Tunnel:Temp:Inlet_Av" {
          w633 = 0.0 ("Value")
          w627 = "EnFlo_Tunnel:Temp:Inlet"
          n219 = String Length(string=w627) -> (length=w628:i32)
          n220 = for {
            tunnel: w635 -> [w641] mode=indexing
            tunnel: w634 -> [w640] mode=indexing
            shift-right: [w648] -> w632
            shift-left: w633 -> [w647]
            shift-right: [w645] -> w631
            shift-left: w633 -> [w646]
            tunnel: w628 -> [w644]
            tunnel: w627 -> [w642]
            tunnel: "EnFlo_Tunnel:Temp:Inlet_Av" -> [w639]
            n221 = String Subset(string=w640, length (rest)=w644) -> (substring=w643:string)  [unwired: 1 out]
            n222 = Equal?(x=w643, y=w642) -> (x = y?=w637:bool)
            n223 = Not Equal?(x=w640, y=w639) -> (x != y?=w638:bool)
            n224 = And(x=w637, y=w638) -> (x .and. y?=w636:bool)
            n225 = case shown="True" w636 {
              tunnel: [w650 w654] -> w648
              tunnel: w647 -> [w650 w655]
              tunnel: w641 -> [_ w653]
              tunnel: w646 -> [w649 w652]
              tunnel: [w649 w651] -> w645
              frame False {
              }
              frame True {
                n226 = Add(x=w653, y=w655) -> (x+y=w654:dbl)
                n227 = Increment(x=w652) -> (x+1=w651:dbl)
              }
            }
          }
          n228 = Divide(x=w632, y=w631) -> (x/y=w630:dbl)
        }
        frame "EnFlo Lab:labstrat1:Av Temp" {
          w660 = 0.0 ("Value")
          n229 = for {
            tunnel: w664 -> [w676]
            tunnel: w663 -> [w675]
            shift-right: [w672] -> w661
            shift-left: "" -> [w673]
            shift-right: [w670] -> w659
            shift-left: w660 -> [w669]
            shift-right: [w666] -> w658
            shift-left: w660 -> [w667]
            tunnel: string[] ["EnFlo Lab:labstrat1:Z=4.5m", "EnFlo Lab:labstrat1:Z=3.5m", "EnFlo Lab:labstrat1:Z=2.5m", "EnFlo Lab:labstrat1:Z=1.5m", "EnFlo Lab:labstrat1:Z=0.5m"] -> [w665] mode=indexing
            n230 = call "Read_value_of_earlier_Ch.vi"("Desired Ch to Read"=w665, "Ch names"=w675, "Present scan array"=w676) -> ("Value"=w668:dbl, "Scan comment"=w674:string)  [unwired: 1 in]
            n231 = Concatenate Strings(w673, w674) -> (w672:string)
            n232 = Not A Number/Path/Refnum?(number/path/refnum=w668) -> (NaN/Path/Refnum?=w671:bool)
            n233 = case shown="True" w671 {
              tunnel: [w680 w683] -> w670
              tunnel: w669 -> [w681 w683]
              tunnel: w668 -> [w679 _]
              tunnel: w667 -> [w678 w682]
              tunnel: [w677 w682] -> w666
              frame False {
                n234 = Add(x=w679, y=w681) -> (x+y=w680:dbl)
                n235 = Increment(x=w678) -> (x+1=w677:dbl)
              }
              frame True {
              }
            }
          }
          n236 = Divide(x=w659, y=w658) -> (x/y=w657:dbl)
        }
        frame "EnFlo Lab:labstrat1:Delta T" {
          n237 = Build Array("EnFlo Lab:labstrat1:Z=4.5m", "EnFlo Lab:labstrat1:Z=0.5m") -> (w691:string[])
          n238 = call "Read_Earlier_Channels.vi"("Present scan array"=w687, "Ch names"=w688, "Desired Channels"=w691) -> ("Scan comments"=w686:string, "Index 0"=w685:dbl, "Index 1"=w684:dbl)  [unwired: 3 out]
          n239 = Subtract(x=w685, y=w684) -> (x-y=w692:dbl)
        }
        frame "Laser:Cooling_Water:Delta_T" {
          n240 = Build Array("LDA Laser:Cooling water:Return Temp", "LDA Laser:Cooling water:Supply Temp") -> (w700:string[])
          n241 = call "Read_Earlier_Channels.vi"("Present scan array"=w696, "Ch names"=w697, "Desired Channels"=w700) -> ("Scan comments"=w695:string, "Index 0"=w694:dbl, "Index 1"=w693:dbl)  [unwired: 3 out]
          n242 = Subtract(x=w694, y=w693) -> (x-y=w701:dbl)
        }
        frame "EnFlo_Tunnel:Chilled Water:Valve Dem Pos" {
          n243 = Get Date/Time In Seconds() -> (seconds since 1Jan1904=w703:timestamp)
          n244 = Concatenate Strings(w704, " last updated") -> (w712:string)
          n245 = To Double Precision Float(number=w703) -> (double precision float=w702:dbl)
          n246 = Unbundle By Name(w710) -> ("A"=w709:dbl)
          n247 = call "Remember_value.vi"("Mode"=Remember_value_mode."Read only", "Ch name"=w712) -> ("Output Value"=w711:dbl)  [unwired: 1 in]
          n248 = Subtract(x=w702, y=w711) -> (x-y=w708:dbl)
          n249 = Greater?(x=w708, y=w709) -> (0:w707:bool)
          n250 = Not A Number/Path/Refnum?(number/path/refnum=w708) -> (NaN/Path/Refnum?=w706:bool)
          n251 = Or(x=w706, y=w707) -> (x .or. y?=w705:bool)
          n252 = case shown="True" w705 {
            tunnel: w719 -> [w720 w739]
            tunnel: [w720 w738] -> w718
            tunnel: w717 -> [_ w730]
            tunnel: w716 -> [_ w731]
            tunnel: ["" w736] -> w715
            tunnel: w712 -> [_ w726]
            tunnel: w702 -> [_ w722]
            frame False {
            }
            frame True {
              n253 = call "Read_value_of_earlier_Ch.vi"("Desired Ch to Read"="EnFlo_Tunnel:Chiller_Pump:Enable", "Ch names"=w731, "Present scan array"=w730) -> ("Value"=w729:dbl)  [unwired: 1 in, 1 out]
              n254 = Build Array("EnFlo_Tunnel:Chilled Water:Dem Temp", "EnFlo_Tunnel:Chilled Water:Supply", "EnFlo_Tunnel:Chiller_Pump:Running") -> (w737:string[])
              n255 = call "Read_Earlier_Channels.vi"("Present scan array"=w730, "Ch names"=w731, "Desired Channels"=w737) -> ("Scan comments"=w736:string, "Index 0"=w735:dbl, "Index 1"=w734:dbl, "Index 2"=w724:dbl)  [unwired: 2 out]
              n256 = Greater?(x=w729, y=0.5) -> (0:w727:bool)
              n257 = Greater?(x=w724, y=0.5) -> (0:w723:bool)
              n258 = case shown="False" w723 {
                tunnel: w739 -> [_ w767]
                tunnel: [w754 w761] -> w738
                tunnel: w735 -> [_ w763]
                tunnel: w734 -> [_ w762]
                tunnel: w722 -> [_ w760]
                tunnel: w727 -> [w745 _]
                tunnel: w726 -> [_ w759]
                frame False {
                  n259 = Seconds To Date/Time() -> (date time rec=w742:T13)  [unwired: 2 out]
                  n260 = Unbundle By Name(w742) -> ("day of week"=w749:i32, "hour"=w751:i32)
                  n261 = Less?(x=w751, y=3) -> (x < y?=w746:bool)
                  n262 = Equal?(x=7, y=w749) -> (x = y?=w747:bool)
                  n263 = And(x=w747, y=w746) -> (x .and. y?=w744:bool)
                  n264 = case shown="True" w745 {
                    tunnel: w744 -> [w755 w757]
                    tunnel: [w755 w756] -> w743
                    frame False {
                    }
                    frame True {
                      n265 = Not(x=w757) -> (.not. x?=w756:bool)
                    }
                  }
                  n266 = Select(t=0.0, s=w743, f=100.0) -> (s? t:f=w754:dbl)
                }
                frame True {
                  w765 = 100.0  # Max
                  w766 = 0.0  # Min
                  n267 = call "PID.vi"("Present Value"=w762, "Previous Control Sum"=w767, "Setpoint"=w763) -> ("Dem Output"=w764:dbl)
                  n268 = In Range and Coerce(upper limit=w765, x=w764, lower limit=w766) -> (coerced(x)=w761:dbl)  [unwired: 1 out]
                  n269 = call "Remember_value.vi"("Mode"=Remember_value_mode."Read and Write", "Input Value"=w760, "Ch name"=w759) -> ()  [unwired: 1 out]
                }
              }
            }
          }
        }
        frame "EnFlo_Tunnel:Hydrosonic:Integral" {
          n270 = Build Array("EnFlo_Tunnel:Usonic Fixed:Velocity", "Hydrosonic:Transducer:Setting") -> (w777:string[])
          n271 = call "Read_Earlier_Channels.vi"("Present scan array"=w778, "Ch names"=w776, "Desired Channels"=w777) -> ("Scan comments"=w770:string, "Index 0"=w775:dbl, "Index 1"=w769:dbl)  [unwired: 3 out]
          n272 = Greater?(x=w775, y=0.5) -> (0:w773:bool)
          n273 = case shown="True" w773 {
            tunnel: w772 -> [w781 w789]
            tunnel: [w781 w788] -> w771
            tunnel: w769 -> [_ w787]
            tunnel: w768 -> [_ w786]
            frame False {
            }
            frame True {
              w784 = 8640000.0  # Seconds per day x 100
              n274 = Multiply(x=w787, y=w786) -> (x*y=w785:dbl)
              n275 = Divide(x=w785, y=w784) -> (x/y=w783:dbl)
              n276 = Not A Number/Path/Refnum?(number/path/refnum=w783) -> (NaN/Path/Refnum?=w782:bool)
              n277 = case shown="False" w782 {
                tunnel: w789 -> [w792 w793]
                tunnel: [w791 w793] -> w788
                tunnel: w783 -> [w790 _]
                frame False {
                  n278 = Add(x=w790, y=w792) -> (x+y=w791:dbl)
                }
                frame True {
                }
              }
            }
          }
        }
        frame "EnFlo_Tunnel:Days Run at:2.5m/s" {
          n279 = Build Array("EnFlo_Tunnel:Usonic Fixed:Velocity") -> (w802:string[])
          n280 = call "Read_Earlier_Channels.vi"("Present scan array"=w803, "Ch names"=w801, "Desired Channels"=w802) -> ("Scan comments"=w796:string, "Index 0"=w794:dbl)  [unwired: 4 out]
          n281 = Greater?(x=w794, y=0.5) -> (0:w799:bool)
          n282 = case shown="True" w799 {
            tunnel: w798 -> [w805 w813]
            tunnel: [w805 w812] -> w797
            tunnel: w794 -> [_ w811]
            tunnel: w795 -> [_ w810]
            frame False {
            }
            frame True {
              w808 = 216000.0  # Seconds per day x 2.5
              n283 = Multiply(x=w811, y=w810) -> (x*y=w809:dbl)
              n284 = Divide(x=w809, y=w808) -> (x/y=w807:dbl)
              n285 = Not A Number/Path/Refnum?(number/path/refnum=w807) -> (NaN/Path/Refnum?=w806:bool)
              n286 = case shown="True" w806 {
                tunnel: w813 -> [w816 w817]
                tunnel: [w815 w817] -> w812
                tunnel: w807 -> [w814 _]
                frame False {
                  n287 = Add(x=w814, y=w816) -> (x+y=w815:dbl)
                }
                frame True {
                }
              }
            }
          }
        }
        frame "Complete:Scan:Period" {
          n288 = while {
            tunnel: [w827] -> w820
            tunnel: [w834] -> w822
            shift-left: _ -> [w834]
            shift-right: [w835] -> w823
            tunnel: w819 -> [w831]
            tunnel: [w826] -> w818
            stop <- FALSE continue-if-true
            w826 = 10.0 ("Averaging time (mins)")
            n289 = Build Array(w831) -> (w830:string[])
            n290 = call "Get_Channel_averages.vi"("Desired Ch Names"=w830, "Averaging time (mins)"=w826) -> ("number"=w829:dbl[])  [unwired: 1 in, 2 out]
            n291 = Index Array(array=w829, index=0) -> (element=w827:dbl)
            n292 = Greater?(x=w827, y=20.0) -> (0:w835:bool)
          }
          n293 = Compound Arithmetic op=AND(w823, invert w822) -> (w821:bool)
          n294 = case shown="True" w821 {
            tunnel: w820 -> [_ w841]
            tunnel: w818 -> [_ w836]
            frame False {
            }
            frame True {
              n295 = Format Into String(format string="Warning! The average scan period on the ADAM Scan table is %.1f seconds over the last %d minutes." ("Format String"), w841, w836) -> (resulting string=w839:string)  [unwired: 2 in, 1 out]
              n296 = call "Server_Emails.vi"("Message"=w839, "Contact All clients?"=TRUE, "Subject"="Scan Period") -> ()  [unwired: 2 in, 3 out]
            }
          }
        }
        frame "GMU:Source:Est Time" {
          # "NaN's"
          # "Est?"
          # "Inband?"
          n297 = stacked-sequence {
            seq-local: [w848 _ _ _] -> [_ _ w895 _]
            seq-local: [_ w860 _ _] -> [_ _ w892 _]
            seq-local: [_ w861 _ _] -> [_ _ w890 _]
            seq-local: [_ _ w897 _] -> [_ _ _ w913]
            seq-local: [w852 _ _ _] -> [_ _ w894 _]
            seq-local: [_ w859 _ _] -> [_ _ _ w909]
            tunnel: w847 -> [w854 w862 w900 _]
            tunnel: w846 -> [w853 w863 w901 _]
            tunnel: [_ _ w893 _] -> w845
            tunnel: [_ _ _ w912] -> w844
            tunnel: w843 -> [_ _ _ w911]
            tunnel: w842 -> [_ _ _ w910]
            frame #0 {
              n298 = Build Array("GMU:Source:Density Ratio", "GMU:Source:Dem Strength", "GMU:Source:Dem Q") -> (w855:string[])
              n299 = call "Read_Earlier_Channels.vi"("Present scan array"=w853, "Ch names"=w854, "Desired Channels"=w855) -> ("Scan comments"=w852:string, "Index 0"=w851:dbl, "Index 1"=w850:dbl, "Index 2"=w849:dbl)  [unwired: 2 out]
              n300 = Build Array(w851, w850, w849) -> (w848:dbl[])
            }
            frame #1 {
              n301 = for {
                N: 2 -> [_]
                tunnel: w863 -> [w873]
                tunnel: w862 -> [w874]
                tunnel: [w872] -> w860 mode=indexing
                tunnel: [w879] -> w861 mode=indexing
                tunnel: [w878] -> w859 mode=indexing
                i -> [w884]
                w883 = 23.0  # %
                n302 = case shown="1" w884 {
                  tunnel: ["GMU:Source:Meas Q" "GMU:Source:Meas Strength"] -> w877
                  tunnel: ["GMU:Source:Dem Q" "GMU:Source:Dem Strength"] -> w876
                  frame 0, Default {
                  }
                  frame 1 {
                  }
                }
                n303 = Build Array(w876, w877) -> (w875:string[])
                n304 = call "Read_Earlier_Channels.vi"("Present scan array"=w873, "Ch names"=w874, "Desired Channels"=w875) -> ("Scan comments"=w872:string, "Index 0"=w870:dbl, "Index 1"=w871:dbl)  [unwired: 3 out]
                n305 = Not A Number/Path/Refnum?(number/path/refnum=w871) -> (NaN/Path/Refnum?=w878:bool)
                n306 = Subtract(x=w871, y=w870) -> (x-y=w869:dbl)
                n307 = Greater Than 0?(x=w870) -> (x > 0?=w880:bool)
                n308 = Less?(x=w869, y=0.05) -> (x < y?=w866:bool)
                n309 = call "In_Range_check.vi"("%"=w883, "Mode"=In_Range."%", "Value"=w871, "Setpoint"=w870) -> ("In Range"=w867:bool)  [unwired: 1 in, 2 out]
                n310 = Or(x=w867, y=w866) -> (x .or. y?=w865:bool)
                n311 = And(x=w865, y=w880) -> (x .and. y?=w881:bool)
                n312 = Compound Arithmetic op=OR(w881, invert w880, w878) -> (w879:bool)
              }
            }
            frame #2 {
              n313 = while {
                tunnel: [w908] -> w896
                tunnel: w895 -> [w907]
                shift-left: _ -> [w908]
                shift-right: [w907] -> _
                stop <- FALSE continue-if-true
              }
              n314 = Equal?(x=w895, y=w896) -> (x = y?=w902:bool)
              n315 = call "Read_value_of_earlier_Ch.vi"("Desired Ch to Read"="GMU:Source:Dem Q", "Ch names"=w900, "Present scan array"=w901) -> ("Value"=w898:dbl)  [unwired: 1 in, 1 out]
              n316 = Greater Than 0?(x=w898) -> (x > 0?=w905:bool)
              n317 = And Array Elements(Boolean array=w890) -> (logical AND=w889:bool)
              n318 = Select(t=w889, s=w905, f=TRUE) -> (s? t:f=w903:bool)
              n319 = Compound Arithmetic op=AND(w902, w903) -> (w897:bool)
              n320 = Concatenate Strings(w892) -> (w891:string)
              n321 = Concatenate Strings(w891, w894) -> (w893:string)
            }
            frame #3 {
              n322 = case shown="True" w913 {
                tunnel: [0.0 w915] -> w912
                tunnel: w911 -> [_ w920]
                tunnel: w910 -> [_ w916]
                tunnel: w909 -> [_ w919]
                frame False {
                }
                frame True {
                  n323 = Or Array Elements(Boolean array=w919) -> (logical OR=w918:bool)
                  n324 = Add(x=w920, y=w916) -> (x+y=w917:dbl)
                  n325 = Select(t=w916, s=w918, f=w917) -> (s? t:f=w915:dbl)
                }
              }
            }
          }
        }
      }
    }
    frame "Hold Value" {
    }
    frame "Read A" {
      n326 = Unbundle By Name(w924) -> ("A"=w923:dbl)
    }
    frame "Read Ch" {
      n327 = Unbundle By Name(w929) -> ("String"=w926:string)
      n328 = call "Read_value_of_earlier_Ch.vi"("Desired Ch to Read"=w926, "Ch names"=w930, "Present scan array"=w931) -> ("Value"=w927:dbl, "Scan comment"=w928:string)  [unwired: 1 in]
    }
    frame "Coded" {
    }
    frame "RetrieveWebpage" {
    }
    frame "Client Info" {
      n329 = global read "ADAM_Global.vi" "Client State Array"() -> (w948:T14[])
      n330 = call "Split_Ch_name.vi"("Ch name"=w942) -> ("Top level"=w940:string, "Low level"=w938:string)  [unwired: 1 out]
      n331 = Equal?(x="Status" ("Substring"), y=w940) -> (x = y?=w939:bool)
      n332 = Select(t=w938, s=w939, f="") -> (s? t:f=w936:string)
      n333 = for {
        tunnel: w948 -> [w957] mode=indexing
        tunnel: [w956] -> w949 mode=indexing
        n334 = Unbundle By Name(w957) -> ("Client Name"=w956:string)
      }
      n335 = Search 1D Array(1D array=w949, element=w936) -> (index of element=w944:i32)  [unwired: 1 out]
      n336 = Less Than 0?(x=w944) -> (x < 0?=w943:bool)
      n337 = Index Array(array=w948, index=w944) -> (element=w947:T14)
      n338 = case shown="False" w943 {
        tunnel: w947 -> [w952 _]
        tunnel: w936 -> [w951 w954]
        tunnel: [w950 w953] -> w946
        frame False {
          n339 = call "Get_Client_Status_string.vi"("Client State Cluster"=w952, "Client Name"=w951) -> ("Code Value"=w950:dbl)  [unwired: 1 in]
        }
        frame True {
          w953 = 7.0 ("Code Value")
          n340 = call "Remember_value.vi"("Mode"=Remember_value_mode."Read and Write", "Input Value"=w953, "Ch name"=w954) -> ()  [unwired: 1 out]
        }
      }
    }
    frame "Web Client" {
      w967 = 7200.0  # 2 Hours in Seconds
      n341 = Get Date/Time In Seconds() -> (seconds since 1Jan1904=w966:timestamp)
      n342 = Concatenate Strings(w975, ":Last read" ("Substring")) -> (w973:string)
      n343 = To Double Precision Float(number=w966) -> (double precision float=w964:dbl)
      n344 = call "Remember_value.vi"("Mode"=Remember_value_mode."Read only", "Ch name"=w973) -> ("Output Value"=w972:dbl)  [unwired: 1 in]
      n345 = Not A Number/Path/Refnum?(number/path/refnum=w972) -> (NaN/Path/Refnum?=w970:bool)
      n346 = Subtract(x=w964, y=w972) -> (x-y=w978:dbl)
      n347 = Greater?(x=w978, y=1800.0) -> (0:w971:bool)
      n348 = Or(x=w971, y=w970) -> (x .or. y?=w958:bool)
      n349 = case shown="True" w958 {
        frame False {
        }
        frame True {
          n350 = global read "Constants_global.vi" "EnFlo SW Folder"() -> (w981:path)
          n351 = Build Path(base path=w981, name or relative path=path "ADAM Server/Sub VI's/Web_Client.vi") -> (appended path=w980:path)
          n352 = Open VI Reference(vi path=w980) -> (vi reference=w985:refnum<vi>, error out=w986:errorcluster)  [unwired: 1 in, 4 out]
          n353 = property class="VI"(reference=w985, error in=w986) -> (reference out=w988:refnum<vi>, error out=w989:errorcluster, "Front Panel Window:Open"=w987:bool)
          n354 = case shown="False" w987 {
            tunnel: w988 -> [w995 w998]
            tunnel: w989 -> [w994 w997]
            tunnel: [w993 w998] -> w990
            tunnel: [w992 w997] -> w991
            frame False {
              n355 = property class="VI"(reference=w995, error in=w994, "Front Panel Window:Open"=TRUE) -> (reference out=w993:refnum<vi>, error out=w992:errorcluster)
            }
            frame True {
            }
          }
          n356 = invoke class="VI" method="Run VI"(reference=w990, error in=w991, "Wait until done"=FALSE, "Auto Dispose Ref"=TRUE) -> ()  [unwired: 1 in, 5 out]
        }
      }
      n357 = Concatenate Strings(w975, ":value time" ("Substring")) -> (w960:string)
      n358 = call "Remember_value.vi"("Mode"=Remember_value_mode."Read only", "Ch name"=w960) -> ("Output Value"=w965:dbl)  [unwired: 1 in]
      n359 = Subtract(x=w964, y=w965) -> (x-y=w963:dbl)
      n360 = call "Remember_value.vi"("Mode"=Remember_value_mode."Read only", "Ch name"=w975) -> ("Output Value"=w979:dbl)  [unwired: 1 in]
      n361 = Greater?(x=w963, y=w967) -> (0:w969:bool)
      n362 = case shown="True" w969 {
        tunnel: w963 -> [_ w1004]
        tunnel: ["" w1002] -> w968
        frame False {
        }
        frame True {
          n363 = Divide(x=w1004, y=3600.0) -> (x/y=w1001:dbl)
          n364 = Format Into String(format string="Value is %d hours old." ("Format String"), w1001) -> (resulting string=w1002:string)  [unwired: 2 in, 1 out]
        }
      }
    }
    frame "X10" {
      (unwired) 1 items=["-----", "A", "B", "C", "D", "E", "F", "G", "H", "I", "J", "K", "L", "M", "N", "O", "P"] ("House Code")
      n365 = Greater Than 0?(x=w1009) -> (x > 0?=w1008:bool)
      n366 = Unbundle By Name(w1014) -> ("Port Name"=w1011:string, "Main"=w1012:i32, "Ch."=w1013:i32)
      n367 = call "X10control.vi"("Port Name"=w1011, "Power Request (ON)"=w1008, "House Code"=w1012, "Unit No."=w1013) -> ()  [unwired: 6 out]
      n368 = Select(t=1.0, s=w1008, f=0.0) -> (s? t:f=w1005:dbl)
    }
    frame "LPA" {
      # "LPA was, IIRC, a serially-polled weighing platform we rented at Surrey for Athena Scaperdas' project at Atkins to weigh a helicopter with rotor running. \nTo add to the fun, it was RS232, so to make it addressable it was polled through an addressable ADAM 485-232 module"
      n369 = call "LPA400_get_rdg.vi"("Channel Name"=w1017, "Address"=w1018) -> ("Output"=w1015:dbl, "Status note"=w1016:string)  [unwired: 4 out]
    }
    frame "ScanPacer" {
      # "Uses a metronome to slow an otherwise over-fast scan table"
      n370 = call "ADAMPacer.vi"("Ch Description"=w1021) -> ("Scan comment"=w1019:string, "Output"=w1020:dbl)  [unwired: 7 in]
    }
    frame "Test" {
      w1025 = 0.0005  # y
      n371 = Get Date/Time In Seconds() -> (seconds since 1Jan1904=w1022:timestamp)
      n372 = To Double Precision Float(number=w1022) -> (double precision float=w1027:dbl)
      n373 = Subtract(x=w1027, y=2969882881.0) -> (x-y=w1026:dbl)
      n374 = Multiply(x=w1026, y=w1025) -> (x*y=w1023:dbl)
      n375 = Random Number (0-1)() -> (number: 0 to 1=w1024:dbl)
      n376 = Add(x=w1024, y=w1023) -> (x+y=w1030:dbl)
    }
    frame "Oops", Default {
    }
  }
  "Output" <- w8
  "Scan comment" <- w5
